vi "First.vi"(8 "Error In":errorcluster, 10 "Known Host In":refnum<class "KnownHost.lvclass">, 11 "KnownHosts In":refnum<class "KnownHosts.lvclass">) -> (0 "Error Out":errorcluster, 1 "Result":T1, 2 "Known Host Out":refnum<class "KnownHost.lvclass">, 3 "KnownHosts Out":refnum<class "KnownHosts.lvclass">)   [LabVIEW 2017, in "Toolkit.lvlib" / "KnownHosts.lvclass"]
uses:
  KnownHosts.lvclass
  KnownHost/KnownHost.lvclass
  Typedefs/Get Results.ctl
  KnownHosts.lvclass/KnownHosts.ctl
  KnownHost/KnownHost.lvclass/KnownHost.ctl
  Toolkit.lvlib
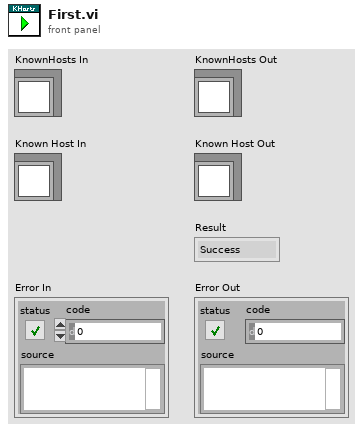
[diagram p1: front panel]
types:
  T1 = typedef "Toolkit.lvlib/KnownHosts.lvclass/Get Results.ctl" = enum32{"Success", "End of Hosts"}
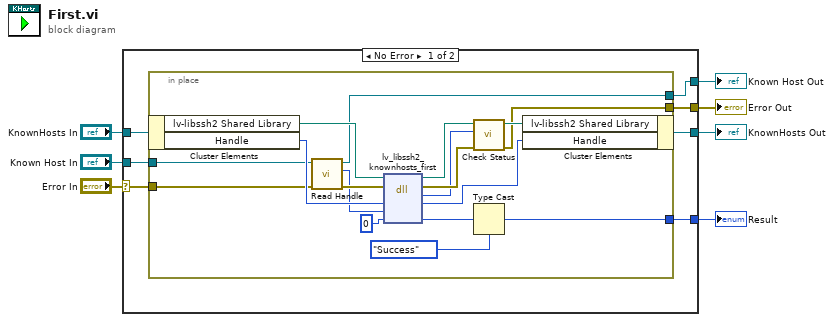
[diagram p0: block diagram]
diagram:
  n1 = case shown="No Error" "Error In" {
    selector: "Error In" -> [w12 w34]
    tunnel: "KnownHosts In" -> [w14 w33]
    tunnel: [w11 w34] -> w5
    tunnel: [w13 w33] -> w4
    tunnel: "Known Host In" -> [w10 w32]
    tunnel: [w9 w32] -> w2
    tunnel: [w8 _] -> w1
    frame No Error {
      n2 = in-place {
        in-place-border: w12 -> [w22]
        in-place-border: [w25] -> w11
        in-place-border: w10 -> [w23]
        in-place-border: [w19] -> w9
        in-place-border: [w15] -> w8
        n3 = in-place-cluster #1(w14) -> ("lv-libssh2 Shared Library"=w29:path, "Handle"=w31:u64)
        n4 = call "Read Handle.vi"("Error In"=w22, "Known Host In"=w23) -> ("Error Out"=w21:errorcluster, "Handle"=w20:u64, "Known Host Out"=w19:refnum<class "KnownHost.lvclass">)  [unwired: 7 in]
        n5 = dll-call lib="lv-libssh2.*" fn="lv_libssh2_knownhosts_first"(path in=w29, error in=w21, "handle"=w31, "host"=w20, "result"=0) -> (path out=w27:path, error out=w28:errorcluster, "status"=w24:i32, "handle"=w30:u64, "result"=w17:i32)  [unwired: 2 in]
        n6 = call "Check Status.vi"("Error In"=w28, "Status"=w24, "lv-libssh2 Shared Library In"=w27) -> ("Error Out"=w25:errorcluster, "lv-libssh2 Shared Library Out"=w26:path)  [unwired: 7 in]
        n7 = Type Cast(type=Get_Results."Success" ("Get Result"), x=w17) -> (*(type *) &x=w15:T1)
        n8 = in-place-cluster #1("lv-libssh2 Shared Library"=w26, "Handle"=w30) -> (w13:refnum<class "KnownHosts.lvclass">)
      }
    }
    frame Error {
    }
  }
  "Error Out" <- w5
  "KnownHosts Out" <- w4
  "Known Host Out" <- w2
  "Result" <- w1
